vi "DoProcess.vi"(8 "error in (no error)":errorcluster, 9 "MsgQ":refnum<queue>, 10 "AbstractionActor.lvclass":refnum<class "AbstractionActor.lvclass">, 11 "UITimeout in":refnum<class "UITimeout.lvclass">) -> (0 "error out":errorcluster, 2 "AbstractionActor.lvclass 2":refnum<class "AbstractionActor.lvclass">, 3 "UITimeout out":refnum<class "UITimeout.lvclass">)   [LabVIEW 2014, in "UITimeout.lvclass"]
uses:
  UITimeout.lvclass
  RealWorkActor/RealWorkActor.lvclass
  AbstractionMessage/AbstractionMessage.lvclass
  AbstractionActor/AbstractionActor.lvclass
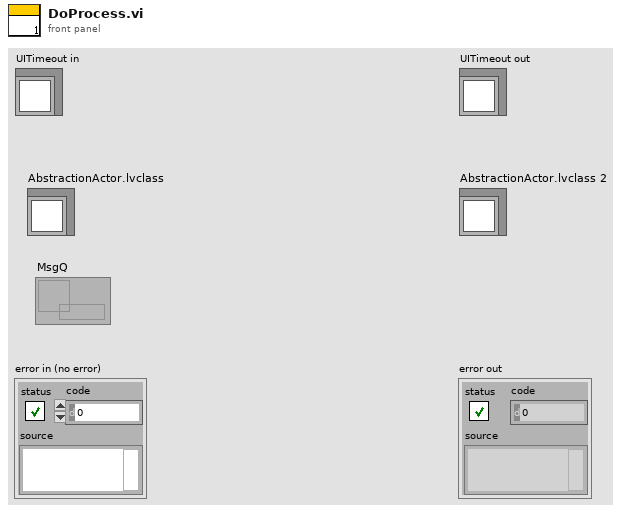
[diagram p1: front panel]
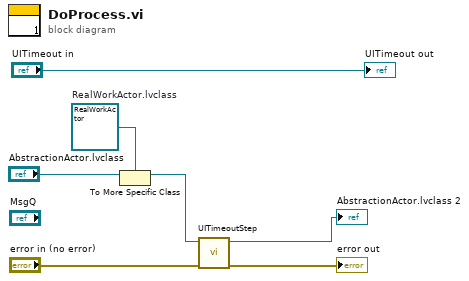
[diagram p0: block diagram]
diagram:
  w1 = refnum<class "RealWorkActor.lvclass"> refnum  # RealWorkActor.lvclass
  n1 = To More Specific Class(target class=w1, reference="AbstractionActor.lvclass") -> (specific class reference=w2:refnum<class "RealWorkActor.lvclass">)  [unwired: 1 in, 1 out]
  n2 = call "UITimeoutStep.vi"("error in (no error)"="error in (no error)", "RealWorkActor in"=w2) -> ("error out"=→"error out":errorcluster, "RealWorkActor out"=→"AbstractionActor.lvclass 2":refnum<class "RealWorkActor.lvclass">)  [unwired: 8 in]
  "UITimeout out" <- "UITimeout in"
